vi "spec_PopulateComboBoxControl.vi"(8 "error in (no error)":errorcluster, 10 "Combo Box Reference":refnum<vi>, 11 "LightField Automation in":refnum<class "LightField Automation.lvclass">) -> (0 "error out":errorcluster, 3 "LightField Automation out":refnum<class "LightField Automation.lvclass">)   [LabVIEW 2018, in "LightField Automation.lvclass"]
uses:
  LightField Automation.lvclass
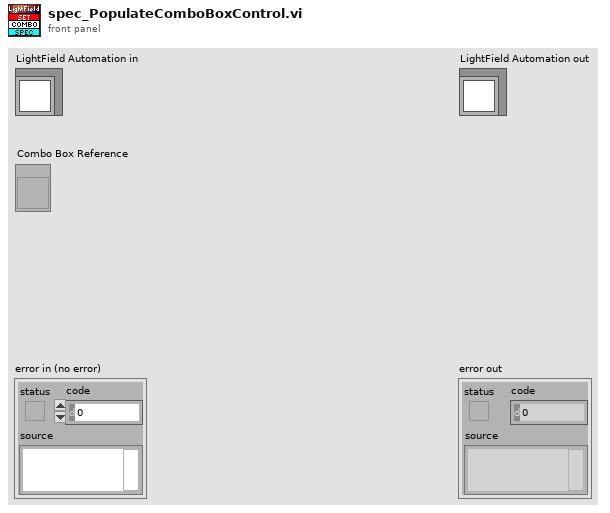
[diagram p1: front panel]
types:
  T1 = cluster{"Parsed Text":string, "GratingSelected":string}[]
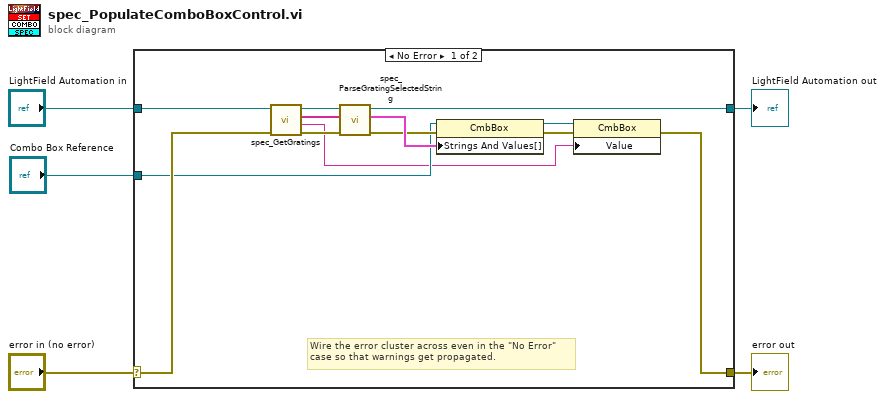
[diagram p0: block diagram]
diagram:
  n1 = case shown="No Error" "error in (no error)" {
    selector: "error in (no error)" -> [w13 w20]
    tunnel: [w6 w20] -> w4
    tunnel: [w14 w19] -> w2
    tunnel: "LightField Automation in" -> [w18 w19]
    tunnel: "Combo Box Reference" -> [w10 _]
    frame No Error {
      # "Wire the error cluster across even in the \"No Error\"\ncase so that warnings get propagated."
      n2 = call "spec_GetGratings.vi"("error in (no error)"=w13, "LightField Automation in"=w18) -> ("error out"=w17:errorcluster, "Current Grating"=w7:string, "Gratings"=w16:string[], "LightField Automation out"=w15:refnum<class "LightField Automation.lvclass">)  [unwired: 6 in]
      n3 = call "spec_ParseGratingSelectedString.vi"("error in (no error)"=w17, "GratingsSelected"=w16, "LightField Automation in"=w15) -> ("error out"=w11:errorcluster, "Strings and Values Array"=w12:T1, "LightField Automation out"=w14:refnum<class "LightField Automation.lvclass">)  [unwired: 6 in]
      n4 = property class="CmbBox"(reference=w10, error in=w11, "Strings And Values[]"=w12) -> (reference out=w9:refnum<vi>, error out=w8:errorcluster)
      n5 = property class="CmbBox"(reference=w9, error in=w8, "Value"=w7) -> (error out=w6:errorcluster)  [unwired: 1 out]
    }
    frame Error {
    }
  }
  "error out" <- w4
  "LightField Automation out" <- w2
